vi "SignalTrap.vi"(11 "Signal":T1) -> (3 "Trapped Signal":bool)   [LabVIEW 2011]
uses:
  Signal.ctl
  SignalAction.ctl
panel:
  # "Signal Traps allow the calling VI to catch a signal\nEach instance owns it's own trap, so all signal traps can catch new signals"
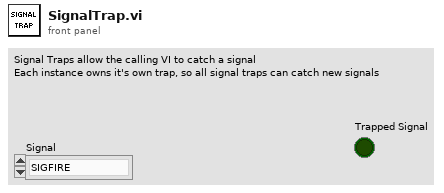
[diagram p1: front panel]
types:
  T1 = typedef "Signal.ctl" = enum16{"SIGFIRE", "SIGSTOPSCRIPT", "SIGSTARTGUN", "SIGSTOPGUN", "SIGDISABLED", "SIGENABLED", "SIGUDPTIMEOUT", "SIGNEWVISION_REMOTE", "SIGNEWVISION_LOCAL", "SIGSHOTFIRED", "SIGDOTRACK", "SIGDONTTRACK"}
  T2 = typedef "SignalAction.ctl" = enum16{"Send Signal", "Get Signal Trap"}
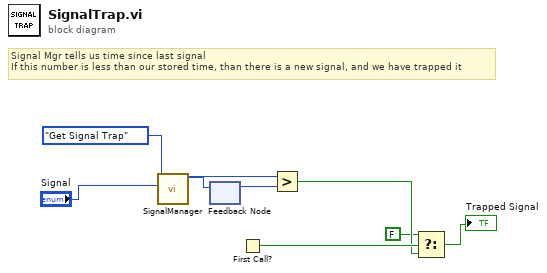
[diagram p0: block diagram]
diagram:
  # "Signal Mgr tells us time since last signal\nIf this number is less than our stored time, than there is a new signal, and we have trapped it"
  n1 = call "SignalManager.vi"("Signal"="Signal", "Signal Action"=SignalAction."Get Signal Trap") -> ("Signal Time"=w6:u32)  [unwired: 9 in]
  n2 = feedback-in #1(w6) -> ()
  n3 = feedback #1() -> (w5:u32)  [unwired: 1 in]
  n4 = First Call?() -> (First Call?: T/F=w4:bool)
  n5 = Greater?(x=w6, y=w5) -> (0:w3:bool)
  n6 = Select(t=FALSE, s=w4, f=w3) -> (s? t:f=→"Trapped Signal":bool)
